vi "Log.vi"(8 "error in (no error)":errorcluster, 10 "Log Text":string, 11 "Sink in":refnum<class "Sink.lvclass">) -> (0 "error out":errorcluster, 3 "Sink out":refnum<class "Sink.lvclass">)   [LabVIEW 2020, in "LV Logging.lvlib" / "Sink.lvclass"]
uses:
  Sink.lvclass
  <vilib>/ErrorRing/Error Ring.xnode
  <vilib>/Utility/error.llb/Error Cluster From Error Code.vi
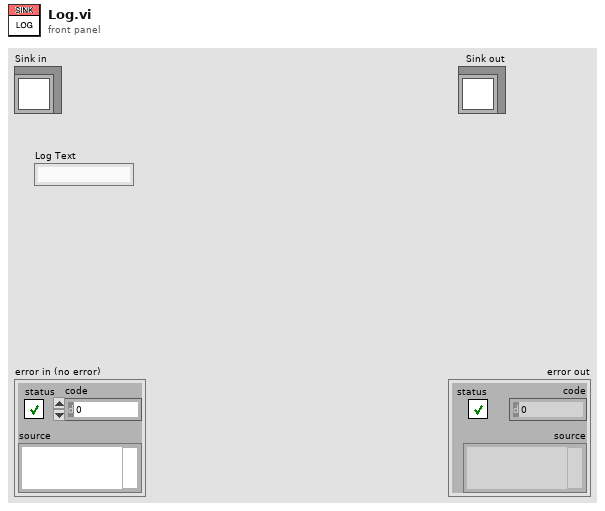
[diagram p1: front panel]
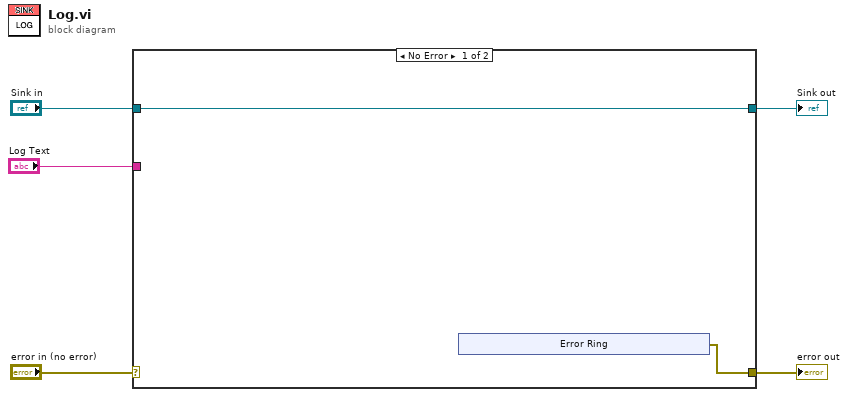
[diagram p0: block diagram]
diagram:
  n1 = case shown="No Error" "error in (no error)" {
    selector: "error in (no error)" -> [_ w14]
    tunnel: [w6 w14] -> w4
    tunnel: [w7 w13] -> w2
    tunnel: "Sink in" -> [w7 w13]
    tunnel: "Log Text" -> [_ _]
    frame No Error {
      n2 = xnode "Error Ring"() -> ("error out"=w6:errorcluster)
    }
    frame Error {
    }
  }
  "error out" <- w4
  "Sink out" <- w2
